vi "backgroundLinearAverageToBRAM.vi"(6 "inputValid":bool, 8 "endOfWave":bool, 9 "startRecording":bool, 10 "bgSatCntP2":u16=12, 11 "input":cluster{"index":u16, "data":i16}) -> (0 "backgroundReady":bool, 3 "bgCount":u16)   [LabVIEW 2016]
uses:
  <vilib>/rvi/Memory/Memory_Emulation/nirvimemoryFastEmulation.vi
  <vilib>/rvi/Memory/Memory_Emulation/nirvimemoryEmulation.vi
  <vilib>/rvi/Emulation/niFpgaEmulationIsFPGAContextNoSignature.vi
  <vilib>/rvi/DataTransferAndStorage/Container/Common/niFpgaContainerGetUniqueNameForEmu.vi
  <vilib>/rvi/Emulation/niFpgaProcessEmulError.vi
  <vilib>/rvi/Emulation/niFpgaSctlEmulationGetInTimedLoop.vi
  <vilib>/rvi/errors/nirviReportUnexpectedCaseInternalError (U32).vi
  <vilib>/rvi/DataTransferAndStorage/Container/XNode/niFpgaContainer.xnode
  <instrlib>/_niInstr/Basic Elements/v1/FPGA/niInstr Basic Elements v1 FPGA.lvlib
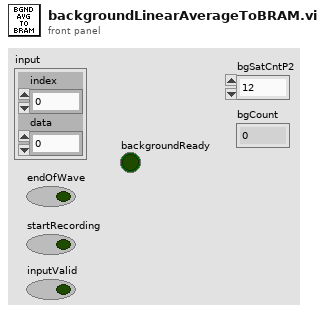
[diagram p1: front panel]
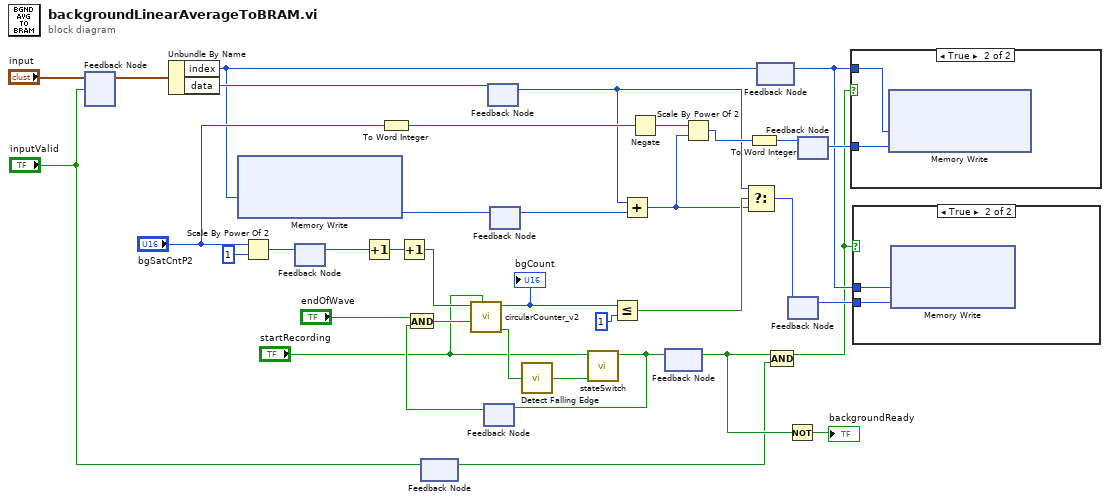
[diagram p0: block diagram]
diagram:
  n1 = feedback-in #1("input", "inputValid") -> ()
  n2 = feedback #1() -> (w4:cluster{"index":u16, "data":i16})  [unwired: 1 in]
  n3 = Unbundle By Name(w4) -> ("index"=w6:u16, "data"=w37:i16)
  n4 = xnode ("Memory Write")("Address"=w6) -> ("Data"=w31:i32)  [unwired: 1 in, 1 out]
  n5 = Scale By Power Of 2(n="bgSatCntP2", x=u16 1) -> (x*2^n=w29:u16)
  n6 = feedback #2() -> (w33:u16)  [unwired: 1 in]
  n7 = feedback-in #2(w29) -> ()
  n8 = Increment(x=w33) -> (x+1=w11:u16)
  n9 = To Word Integer(number="bgSatCntP2") -> (16bit integer=w20:i16)
  n10 = Increment(x=w11) -> (x+1=w15:u16)
  n11 = feedback-in #3("inputValid") -> ()
  n12 = feedback #3() -> (w1:bool)  [unwired: 1 in]
  n13 = feedback #4() -> (w18:bool)  [unwired: 1 in]
  n14 = And(x="endOfWave", y=w18) -> (x .and. y?=w36:bool)
  n15 = call "circularCounter_v2.vi"("reset"="startRecording", "doStep"=w36, "maxCount"=w15) -> ("maxReached"=w19:bool, "index"=w14:u16)  [unwired: 5 in, 2 out]
  "bgCount" <- w14
  n16 = feedback #5() -> (w9:i16)  [unwired: 1 in]
  n17 = feedback-in #5(w37) -> ()
  n18 = feedback #6() -> (w27:i32)  [unwired: 1 in]
  n19 = feedback-in #6(w31) -> ()
  n20 = call <instrlib>:"Detect Falling Edge.vi"("signal"=w19) -> ("edge detected"=w12:bool)  [unwired: 14 in]
  n21 = call "stateSwitch.vi"("disable"=w12, "enable"="startRecording") -> ("state"=w17:bool)  [unwired: 9 in]
  n22 = feedback-in #4(w17) -> ()
  n23 = Less Or Equal?(x=w14, y=u16 1) -> (x <= y?=w35:bool)
  n24 = Add(x=w9, y=w27) -> (x+y=w21:i32)
  n25 = Negate(x=w20) -> (-x=w25:i16)
  n26 = feedback #7() -> (w16:bool)  [unwired: 1 in]
  n27 = feedback-in #7(w17) -> ()
  n28 = Scale By Power Of 2(n=w25, x=w21) -> (x*2^n=w24:i32)
  n29 = Select(t=w9, s=w35, f=w21) -> (s? t:f=w30:i32)
  n30 = To Word Integer(number=w24) -> (16bit integer=w23:i16)
  n31 = feedback-in #8(w6) -> ()
  n32 = feedback #8() -> (w5:u16)  [unwired: 1 in]
  n33 = Compound Arithmetic op=AND(w16, w1) -> (w3:bool)
  n34 = Not(x=w16) -> (.not. x?=→"backgroundReady":bool)
  n35 = feedback #9() -> (w32:i32)  [unwired: 1 in]
  n36 = feedback-in #9(w30) -> ()
  n37 = feedback #10() -> (w22:i16)  [unwired: 1 in]
  n38 = feedback-in #10(w23) -> ()
  n39 = case shown="True" w3 {
    tunnel: w22 -> [_ w39]
    tunnel: w5 -> [_ w38]
    frame False {
    }
    frame True {
      n40 = xnode ("Memory Write")("Address"=w38, "Data"=w39) -> ()  [unwired: 1 in, 1 out]
    }
  }
  n41 = case shown="True" w3 {
    tunnel: w32 -> [_ w41]
    tunnel: w5 -> [_ w40]
    frame False {
    }
    frame True {
      n42 = xnode ("Memory Write")("Address"=w40, "Data"=w41) -> ()  [unwired: 1 in, 1 out]
    }
  }
